vi "Error FGV.vi"(9 "error in":errorcluster, 10 "Set?":bool) -> (1 "error out":errorcluster)   [LabVIEW 2023, in "Adjust FP VIs.lvlib"]
uses:
  Adjust FP VIs.lvlib
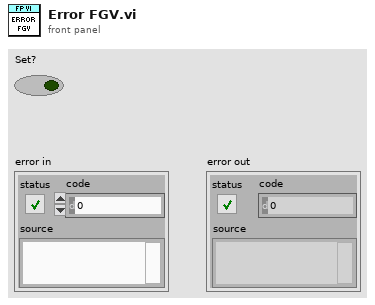
[diagram p1: front panel]
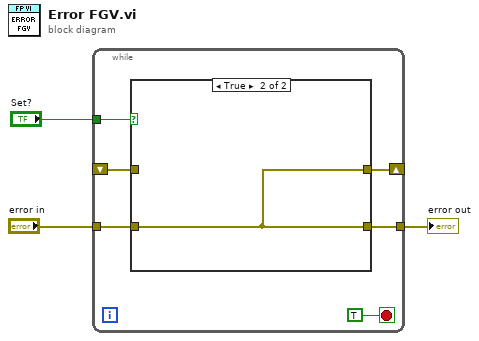
[diagram p0: block diagram]
diagram:
  n1 = while {
    tunnel: "Set?" -> [w8]
    tunnel: "error in" -> [w7]
    shift-right: [w6] -> _
    shift-left: _ -> [w5]
    tunnel: [w4] -> w1
    stop <- TRUE stop-if-true
    n2 = case shown="True" w8 {
      tunnel: w7 -> [_ w11]
      tunnel: [w10 w11] -> w6
      tunnel: w5 -> [w10 _]
      tunnel: [w10 w11] -> w4
      frame False {
      }
      frame True {
      }
    }
  }
  "error out" <- w1
